vi "Start.vi"(7 "Buffer Size (4096)":i32=4096, 8 "error in (no error)":errorcluster, 11 "Mixer in":refnum<class "Mixer.lvclass">) -> (0 "error out":errorcluster, 3 "Mixer out":refnum<class "Mixer.lvclass">)   [LabVIEW 2020, in "G-Audio.lvlib" / "Mixer.lvclass"]
uses:
  Mixer.lvclass
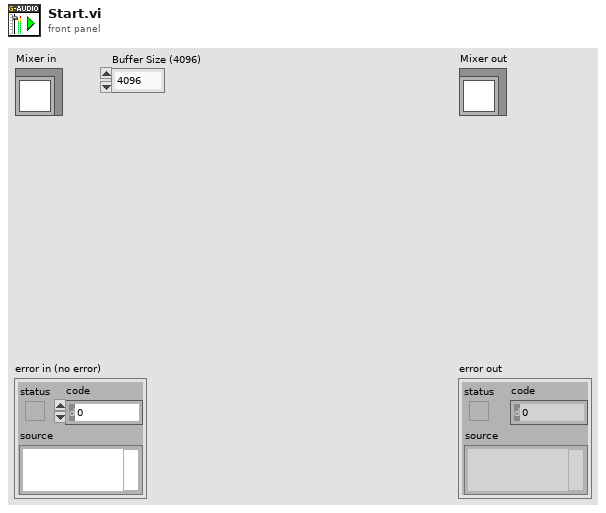
[diagram p1: front panel]
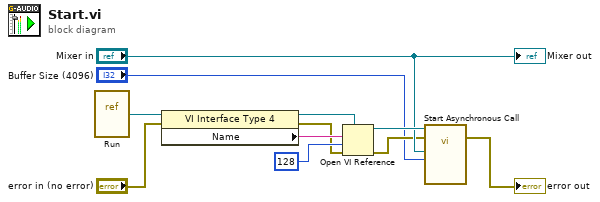
[diagram p0: block diagram]
diagram:
  n1 = vi-ref "Run.vi"() -> (w11:refnum<vi>)
  n2 = property class="VI Interface Type 4"(reference=w11, error in="error in (no error)") -> (reference out=w9:refnum<vi>, error out=w4:errorcluster, "Name"=w10:string)
  n3 = Open VI Reference(type specifier VI Refnum (for type only)=w9, vi path=w10, options=128, error in (no error)=w4) -> (vi reference=w8:refnum<vi>, error out=w3:errorcluster)  [unwired: 2 in]
  n4 = call-by-ref "Start Asynchronous Call"(reference=w8, error in=w3, "Buffer Size"="Buffer Size (4096)", "Mixer in"="Mixer in") -> (error out=→"error out":errorcluster)  [unwired: 8 in, 3 out]
  "Mixer out" <- "Mixer in"
